vi "Dashboard Main.vi"() -> ()   [LabVIEW 2020]
uses:
  <vilib>/event_ctls.llb/eventvkey.ctl
  <vilib>/Rock Robotics/Network Tables/NT Read Boolean.vi
  <vilib>/Rock Robotics/WPI/Dashboard/WPI_DashboardLogging Global.vi
panel:
  out "Background":bool
  in  "Camera Settings Right":T1={"Frame Rate"=30, "Compression"=30, "Size"=1, "DB Camera Config"=FALSE} {"Frame Rate" scale=1.0..30.0; "Compression" scale=100.0..-1.0; "Size" items=["640x480", "320x240", "160x120"]}
  in  "Camera Name Right":string(combo)="No Camera Selection"
  out "Camera Perf":string
  in  "Camera Settings":T1={"Frame Rate"=30, "Compression"=30, "Size"=1, "DB Camera Config"=FALSE} {"Frame Rate" scale=1.0..30.0; "Compression" scale=100.0..-1.0; "Size" items=["640x480", "320x240", "160x120"]}
  in  "TCP":refnum<k5>
  in  "Rec Mode":enum32{"Stop", "Record", "Playback"}(radio)
  out "Robot IP":string
  out "Image Message":string="Timeout in Camera Communications"
  in  "Dashboard Tab":T2(tab)
  out "Shelf":bool
  in  "Select Auto":string(combo)="Select Autonomous ..."
  out "NT Connection":bool
  out "JS1 Z":dbl(slide) scale=-1.0..1.0 scale format="%#_2e"
  out "JS1 Graph":cluster{"X":dbl, "Y":dbl}[](graph)
  out "JS1 Buttons":T3
  out "JS2 Z":dbl(slide) scale=-1.0..1.0 scale format="%#_2e"
  out "JS2 Graph":cluster{"X":dbl, "Y":dbl}[](graph)
  out "JS2 Buttons":T3
  out "Mode":T4(ring)=enum."Auto Disabled"
  out "Right Camera Perf":cluster{"Bandwidth (Mbps)":dbl, "FPS":dbl}
  out "Moving\nto Target":bool
  out "At Target":bool
  out "Arm \nOverride":bool
  out "Top":bool
  out "Middle":bool
  out "Bottom":bool
  out "Game\nPiece":bool
  out "Speed Modifer":dbl
  out "Reverse":bool
  out "Current Action":string
  out "LiftDmd":dbl
  out "ExtendDmd":dbl
  out "Floor":bool
  out "Camera Image Right":T5(plugin-control)
  in  "DB/String 9":string
  in  "DB/String 8":string
  in  "DB/String 7":string
  in  "DB/String 6":string
  in  "DB/String 5":string
  in  "DB/String 4":string
  in  "DB/String 3":string
  in  "DB/String 2":string
  in  "DB/String 1":string
  in  "DB/String 0":string
  in  "DB/Slider 0":dbl(slide) scale=0.0..5.0
  in  "DB/Slider 1":dbl(slide) scale=0.0..5.0
  in  "DB/Slider 2":dbl(slide) scale=0.0..5.0
  in  "DB/Slider 3":dbl(slide) scale=0.0..5.0
  out "DB/LED 3":bool
  out "DB/LED 2":bool
  out "DB/LED 1":bool
  out "DB/LED 0":bool
  in  "DB/Button 3":bool
  in  "DB/Button 2":bool
  in  "DB/Button 1":bool
  in  "DB/Button 0":bool caption="New Name"
  in  "Test Slider":dbl(slide) scale=0.0..100.0 scale format="%#_3g"
  in  "On/Off":bool caption="Solenoid"
  in  "Test Name":u16(ring) items=["Select the test to run..."]
  in  "Test Tree":string(tree)
  in  "Motor":cluster{"Value":dbl, "Enable":bool} {"Value" scale=-1.0..1.0 scale format="%#_3g"}
  out "Progress":T6 {"Test Progress" scale=0.0..100.0}
  in  "Rev/Fwd":cluster{"Forward":bool, "Reverse":bool}
  in  "Test Ring":u16(ring) items=["Monochrome", "Color"]
  in  "CheckList":i32(listbox)
  out "Tree":string(tree)
  out "Camera Image":T5(plugin-control)
  in  "Camera Name":string(combo)="No Camera Selection"
  # "HW"
  # "HW"
  # "Joysticks"
  # "This tab is a great place for autonomous settings and robot-specific values.\nPlace controls and indicators inside this tab and match name to\nDashboard Variables on robot. You can also delete this comment."
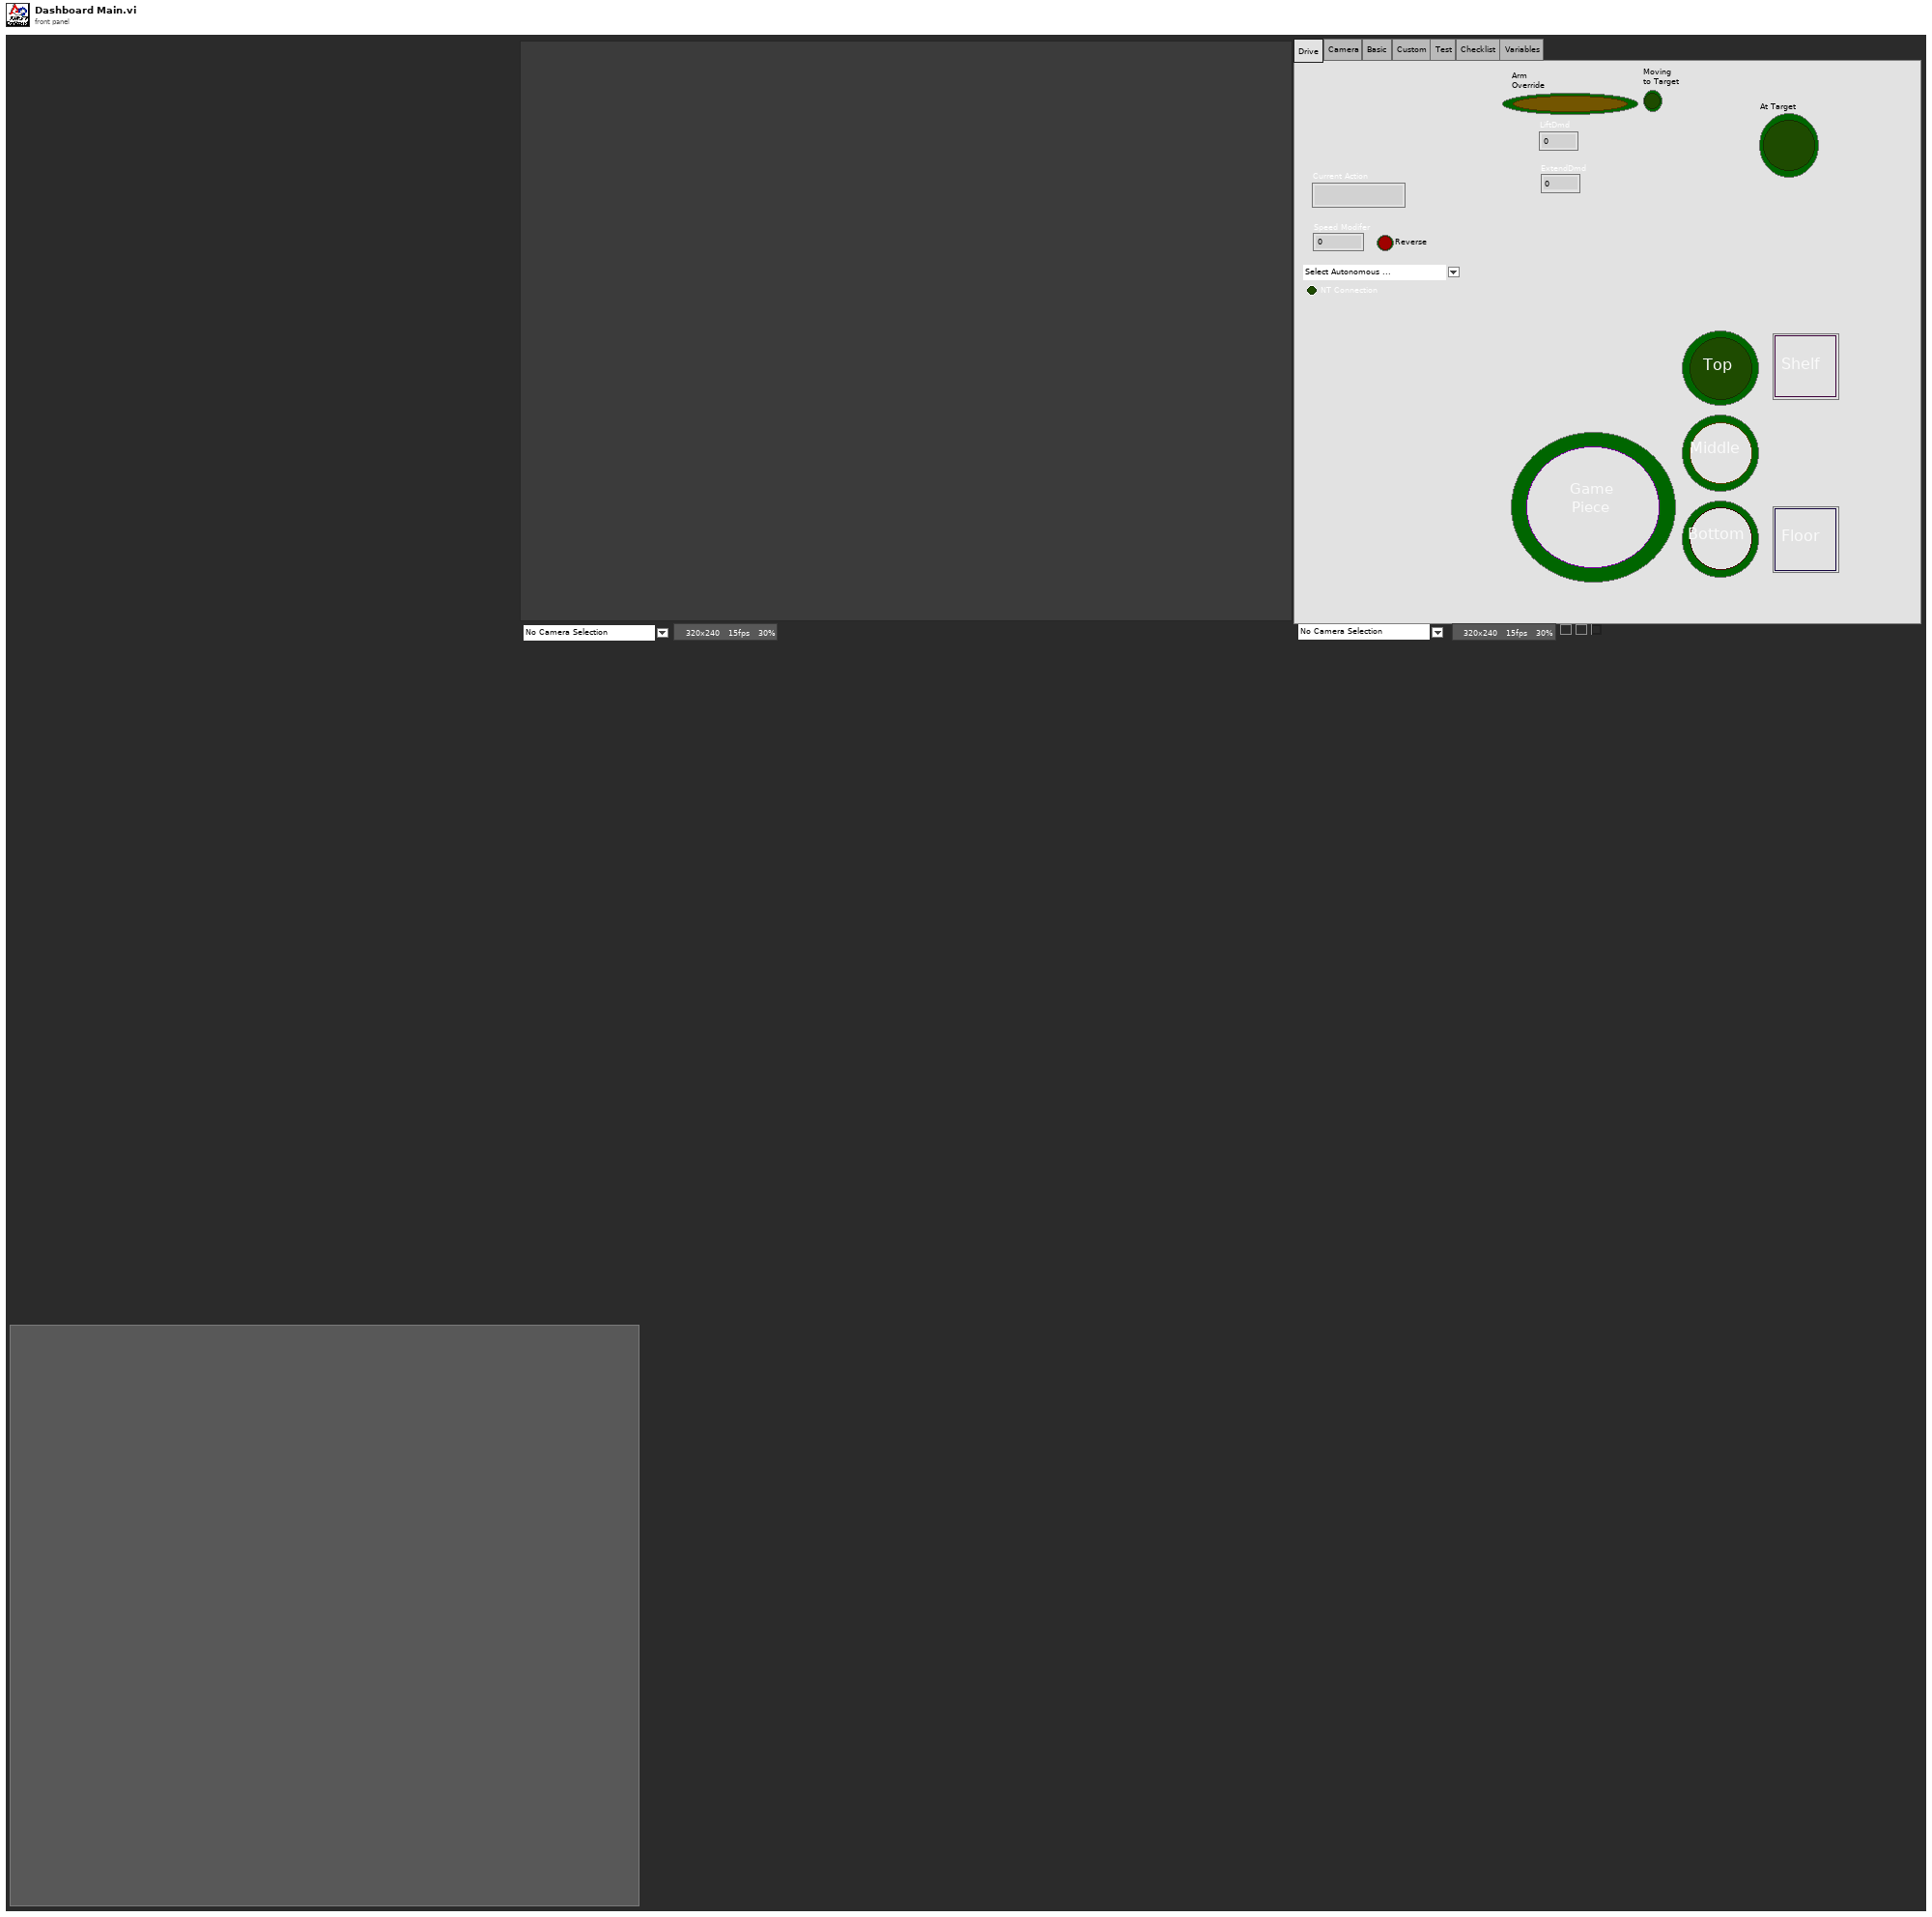
[diagram p1: front panel]
types:
  T1 = cluster{"Frame Rate":i32, "Compression":i32, "Size":u16, "DB Camera Config":bool}
  T2 = enum32{"Drive", "Camera", "Basic", "Custom", "Test", "Checklist", "Variables"}
  T3 = cluster{bool, bool, bool, bool, bool, bool, bool, bool, bool, bool, bool, bool}
  T4 = enum8{"Tele-Op Disabled", "Tele-Op Enabled", "Auto Disabled", "Auto Enabled", "Test Disabled", "Test Enabled", "Disconnected", "No Code", "E-Stop"}
  T5 = typedef "IMAQ Image.ctl" = refnum<image>
  T6 = cluster{"Test Progress":u8, "Test Progress Text":string}
  T7 = cluster{"Save Path":path, "Interval (s)":dbl, "Keep":i32}
  T8 = enum32{"Drive", "Camera", "Basic", "Custom", "Test", "Commands", "Checklist", "Variables"}
  T9 = typedef "Image Type" = u32
  T10 = cluster{"Error Strings":string, "Disable Counts":cluster{u16, u16}, "Rail Faults":cluster{u16, u16, u16}, "Robot IP":string, "DB Mode":u8, "Event Info":cluster{"Name":string, "Type":u8, "Number":u16, "Replay":u8}}
  T11 = cluster{"Storage":cluster{"Disk Free":u64, "RAM Block":u32, "RAM free":u32}, "CPU Utilization":cluster{"CPU % ISR":sgl, "CPU % Time Crit":sgl, "CPU % Timed Str":sgl, "CPU % High":sgl, "CPU % Above":sgl, "CPU % Normal":sgl, "CPU % Low":sgl}, "CAN":cluster{"% Bus Utilization":sgl, "Bus Off Cnt":u32, "TX_FIFO Full Cnt":u32, "Receive Error Cnt":u8, "Transmit Error Cnt":u8}, "HID":cluster{"HID Outputs":u32, "Rumble Low":u16, "Rumble High":u16}[]}
  T12 = cluster{"Status bits":cluster{"Test Mode":bool, "Autonomous":bool, "Enabled":bool, "Code Start":bool, "Brownout":bool, "Reserved 2":bool, "Reserved 3":bool, "E-Stop":bool}, "Code Trace":cluster{"Disabled":bool, "TeleOp":bool, "Auto":bool, "Test":bool}, "Controller Type":enum16{"unknown", "cRIO", "roboRio"}, "Code?":enum16{"unknown", "noCode", "code"}, "Battery V":dbl}
  T13 = cluster{"Control Bits":cluster{"TestMode":bool, "Autonomous":bool, "Enabled":bool, "FMS Present":bool, bool, bool, bool, "E-Stop":bool}, "Team Station ":u8, "Countdown":sgl, "Joystick Values":cluster{"Axes":dbl[], "Buttons":bool[], "POVs":i16[]}[]}
  T14 = cluster{"Axes":dbl[], "Buttons":bool[], "POVs":i16[]}[]
  T15 = cluster{"Axes":dbl[], "Buttons":bool[], "POVs":i16[]}
  T16 = cluster{"Buttons[0]":bool, "Buttons[1]":bool, "Buttons[2]":bool, "Buttons[3]":bool, "Buttons[4]":bool, "Buttons[5]":bool, "Buttons[6]":bool, "Buttons[7]":bool, "Buttons[8]":bool, "Buttons[9]":bool, "Buttons[10]":bool, "Buttons[11]":bool}
  T17 = cluster{"Camera Image":refnum<vi>, "Dashboard Tab":refnum<vi>, "Background":refnum<vi>, "Rec Mode":refnum<vi>, "Test Slider":refnum<vi>, "On/Off ":refnum<vi>, "Test Ring":refnum<vi>, "Rev/Fwd":refnum<vi>, "Test Name":refnum<vi>, "Motor":refnum<vi>, "Progress":refnum<vi>, "CheckList":refnum<vi>, "Tree":refnum<vi>, "Test Tree":refnum<vi>, "Camera Settings":refnum<vi>, "Camera Name":refnum<vi>, "Camera Perf":refnum<vi>, "Camera Settings Right":refnum<vi>, "Camera Name Right":refnum<vi>, "Camera Image Right":refnum<vi>}
  T18 = cluster{"Global Rectangle":i32[], "Contours":cluster{"Contour Type":u32, "ROI Type":u32, "Points":i32[]}[]}
  T19 = cluster{"Camera Name":string, string, "Saved DB Images Info":cluster{"Save Path":path, "Interval (s)":dbl, "Keep":i32}}
  T20 = cluster{"Camera Name Right":string, string, "Saved DB Images Info":cluster{"Save Path":path, "Interval (s)":dbl, "Keep":i32}}
  T21 = cluster{"Operation":enum16{"Update", "Clear"}, "Color Box":u32}[]
  T22 = typedef "eventvkey.ctl" = enum16{"ASCII", "Enter", "Return", "Shift", "Ctrl", "Alt", "Cmd", "Opt", "Caps", "NumLock", "Clear", "Break", "Up", "Down", "Left", "Right", "Insert", "Delete", "Home", "End", "PageUp", "PageDown", "Escape", "Help", "Pause", "ScrollLock", "F1", "F2", "F3", "F4", "F5", "F6", "F7", "F8", "F9", "F10", "F11", "F12", "F13", "F14", "F15", "F16", "F17", "F18", "F19", "F20", "F21", "F22", "F23", "F24", "Play", "VolumeUp", "VolumeDown", "Mute", "Two Byte Char"}
  T23 = cluster{"Image Size":bool, "Image Type":bool, "Pixel Value":bool, "ROI Information":bool, "Zoom Factor":bool}
  T24 = cluster{"Operation":enum16{"Update", "Clear"}, "Color Box":u32}
  T25 = cluster{"Shift":bool, "Ctrl":bool, "Alt":bool, "Cmd":bool, "Opt":bool}
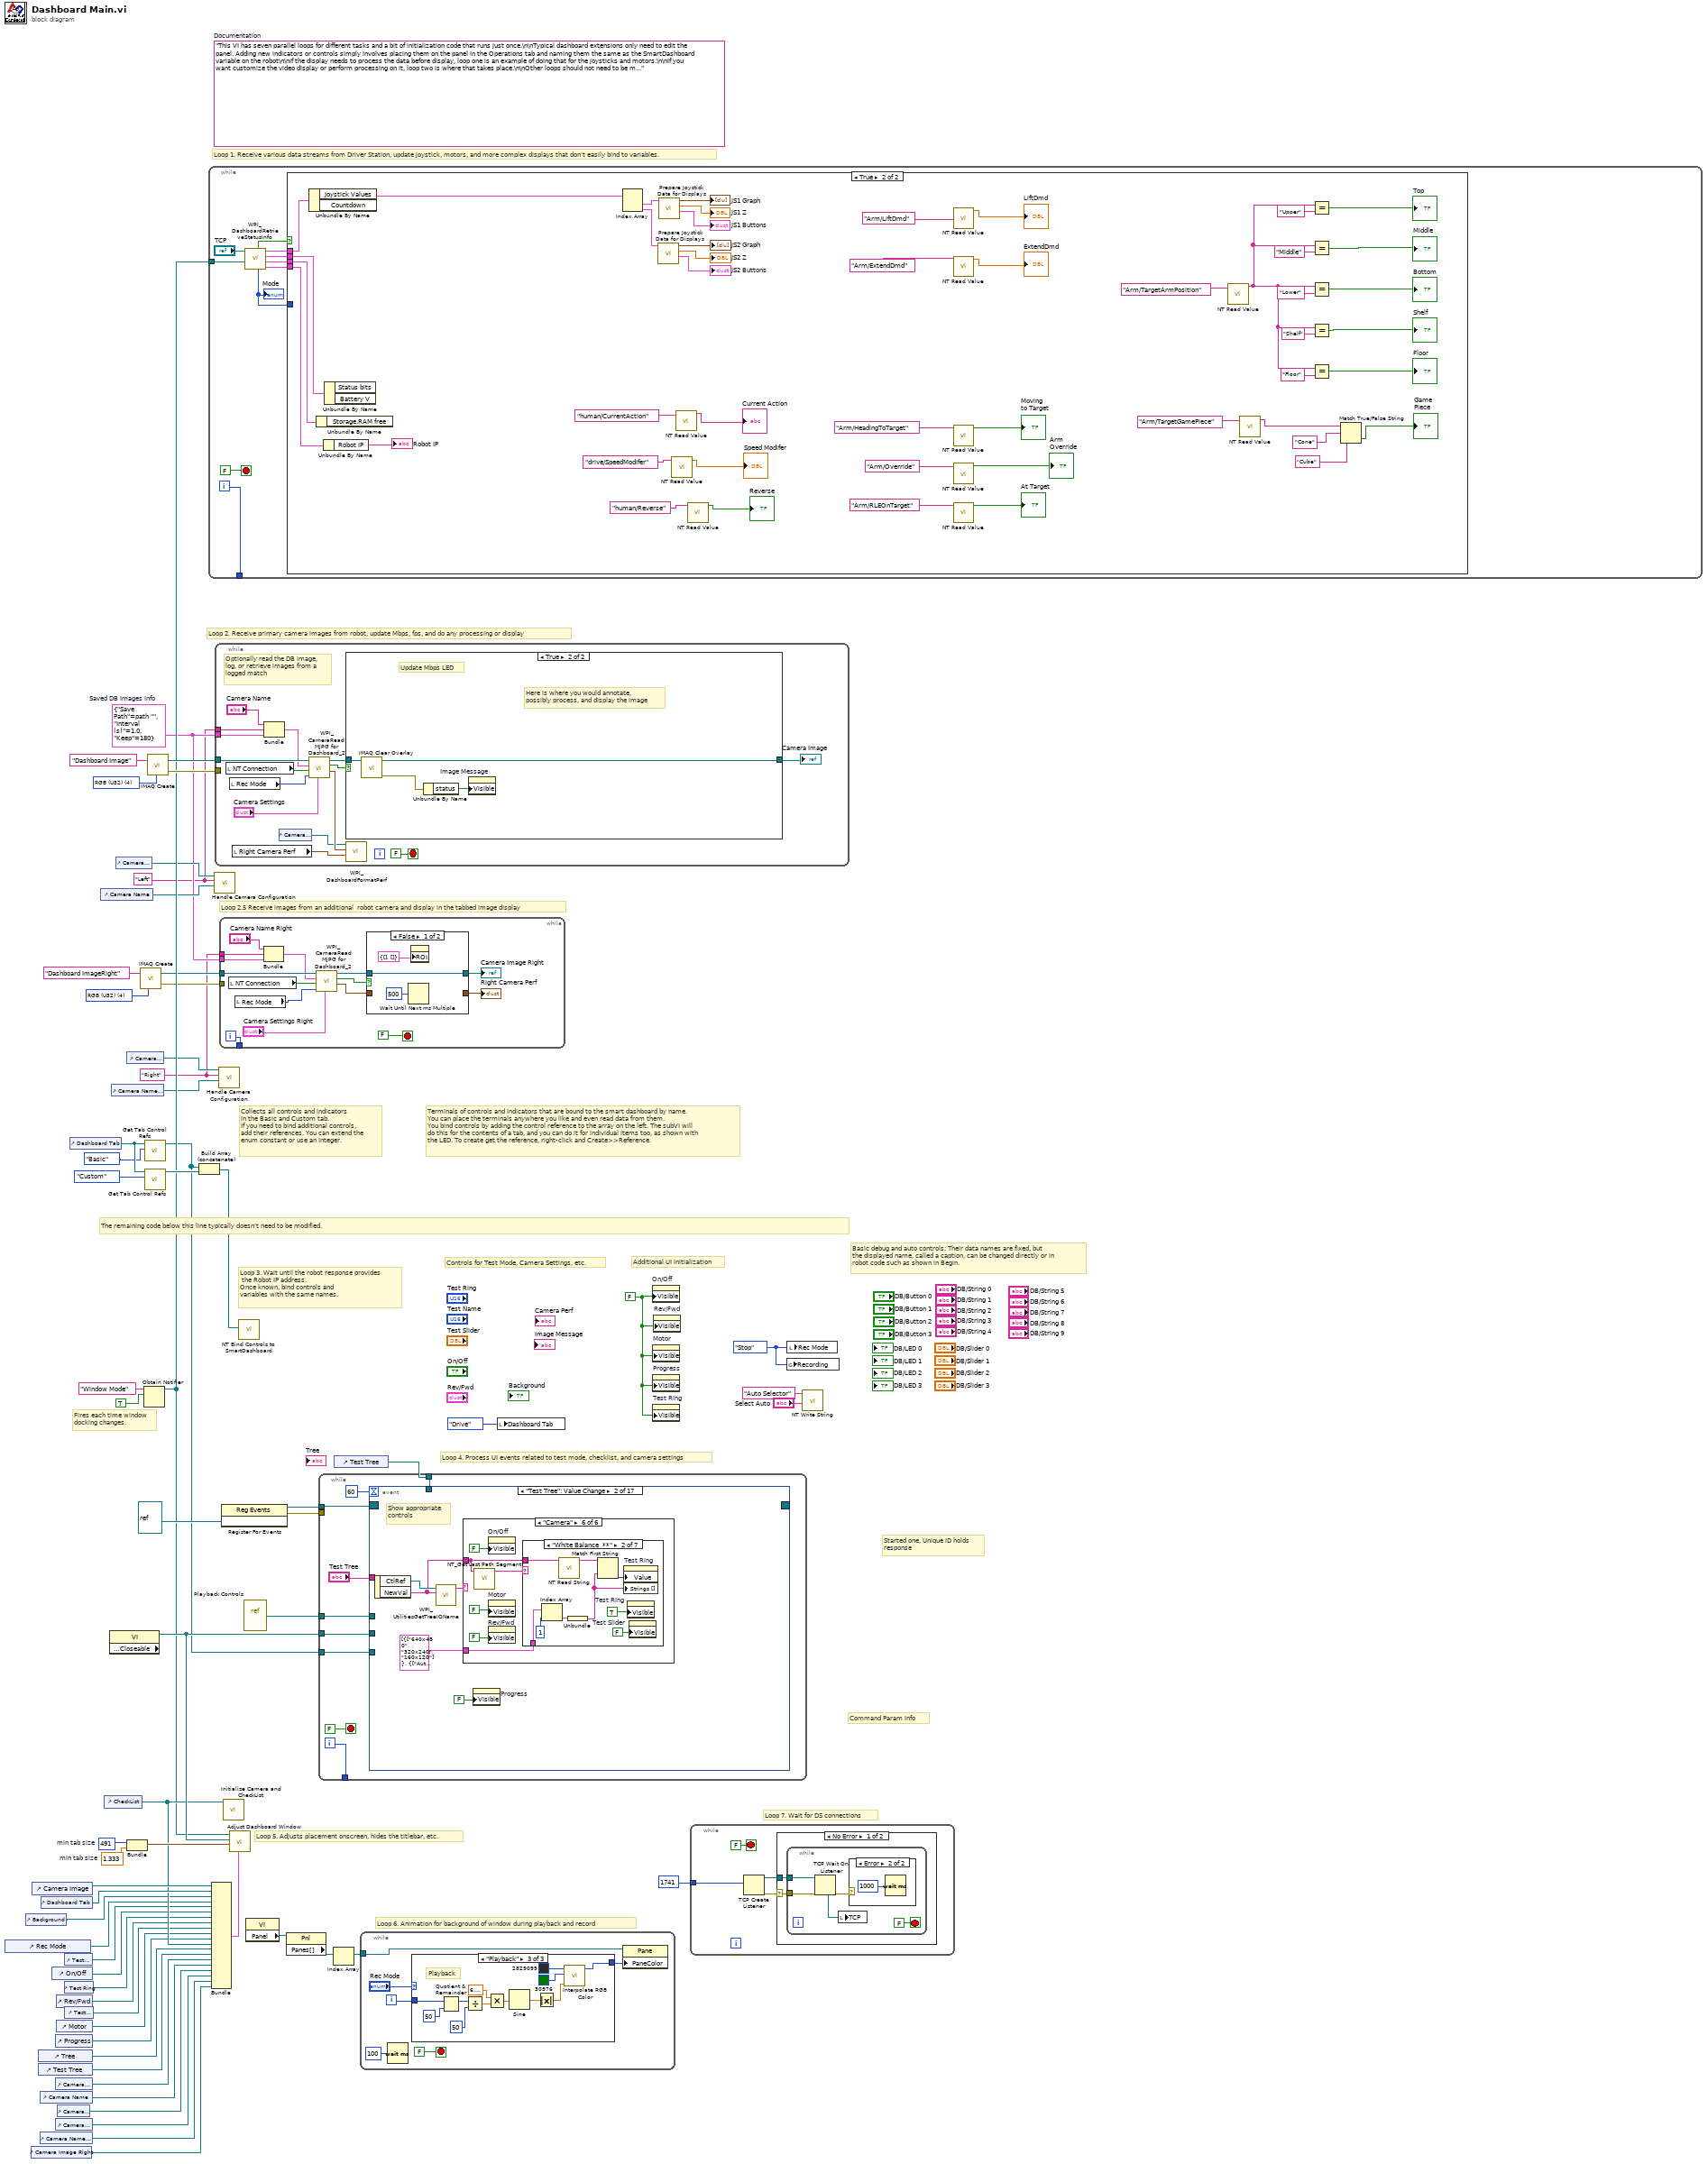
[diagram p0: block diagram]
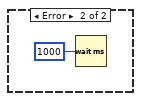
[diagram p4: hidden frame]
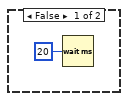
[diagram p5: hidden frame]
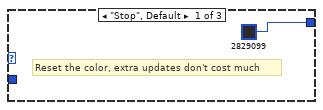
[diagram p6: hidden frame]
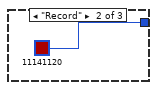
[diagram p7: hidden frame]
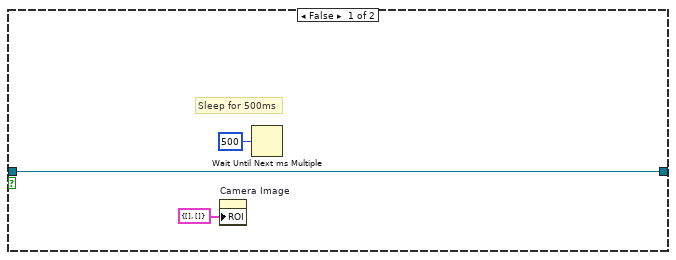
[diagram p8: hidden frame]
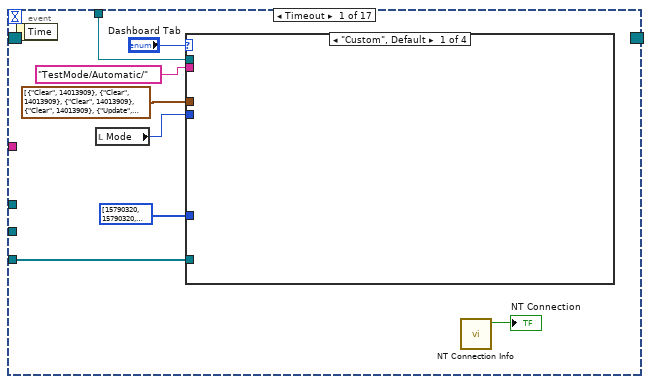
[diagram p9: hidden frame]
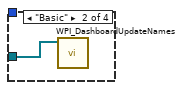
[diagram p10: hidden frame]
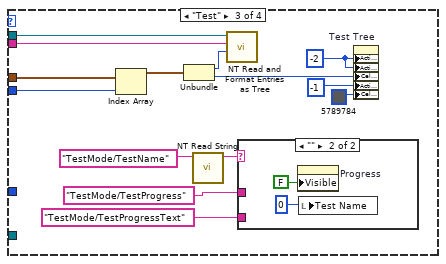
[diagram p11: hidden frame]
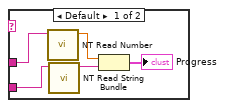
[diagram p12: hidden frame]
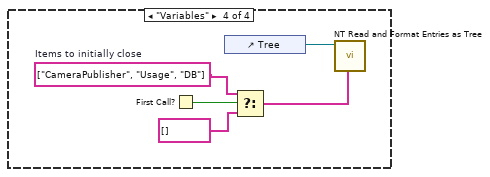
[diagram p13: hidden frame]
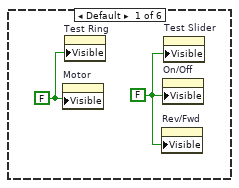
[diagram p14: hidden frame]
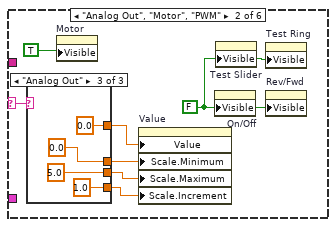
[diagram p15: hidden frame]
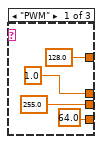
[diagram p16: hidden frame]
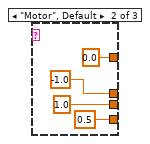
[diagram p17: hidden frame]
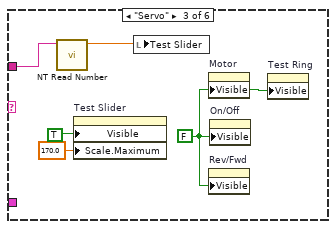
[diagram p18: hidden frame]
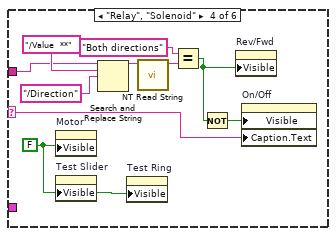
[diagram p19: hidden frame]
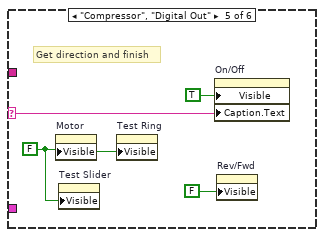
[diagram p20: hidden frame]
diagram:
  w4 = T7 {"Save Path"=path "", "Interval (s)"=1.0, "Keep"=180}  # Saved DB Images Info
  w3 = "Right"
  w2 = "Left"
  w14 = T9 4 items=["Grayscale (U8)", "Grayscale (I16)", "Grayscale (SGL)", "Complex (CSG)", "RGB (U32)", "HSL (U32)", "RGB (U64)"] ("Image Type")
  w42 = 491  # min tab size
  w41 = 1.333  # min tab size
  w49 = enum32{"Stop", "Record", "Playback"}."Stop" ("Rec Mode")
  w27 = FALSE ("Visible")
  (unwired) "This VI has seven parallel loops for different tasks and a bit of initialization code that runs just once.\n\nTypical dashboard extensions only need to edit the panel. Adding new indicators or controls simply involves placing them on the panel in the Operations tab and naming them the same as the SmartDashboard variable on the robot\n\nIf the display needs to process the data before display, loop one is an example of doing that for the joysticks and motors.\n\nIf you want customize the video display or perform processing on it, loop two is where that takes place.\n\nOther loops should not need to be modified. They are pretty standard, and document the task they perform."  # Documentation
  w63 = T9 4 items=["Grayscale (U8)", "Grayscale (I16)", "Grayscale (SGL)", "Complex (CSG)", "RGB (U32)", "HSL (U32)", "RGB (U64)"] ("Image Type")
  # "Loop 2.5 Receive images from an additional  robot camera and display in the tabbed image display"
  # "Command Param Info"
  # "Started one, Unique ID holds\nresponse"
  # "Loop 7. Wait for DS connections"
  # "Basic debug and auto controls: Their data names are fixed, but\nthe displayed name, called a caption, can be changed directly or in\nrobot code such as shown in Begin."
  # "Controls for Test Mode, Camera Settings, etc."
  # "Additional UI Initialization"
  # "Loop 6. Animation for background of window during playback and record"
  # "Fires each time window\ndocking changes."
  # "Collects all controls and indicators\nin the Basic and Custom tab.\nIf you need to bind additional controls,\nadd their references. You can extend the\nenum constant or use an integer."
  # "The remaining code below this line typically doesn't need to be modified."
  # "Loop 4. Process UI events related to test mode, checklist, and camera settings"
  # "Terminals of controls and indicators that are bound to the smart dashboard by name.\nYou can place the terminals anywhere you like and even read data from them.\nYou bind controls by adding the control reference to the array on the left. The subVI will\ndo this for the contents of a tab, and you can do it for individual items too, as shown with\nthe LED. To create get the reference, right-click and Create>>Reference."
  # "Loop 3. Wait until the robot response provides\n the Robot IP address.\nOnce known, bind controls and\nvariables with the same names."
  # "Loop 5. Adjusts placement onscreen, hides the titlebar, etc."
  # "Loop 1. Receive various data streams from Driver Station, update joystick, motors, and more complex displays that don't easily bind to variables."
  # "Loop 2. Receive primary camera images from robot, update Mbps, fps, and do any processing or display"
  n1 = control-ref of="Rec Mode"() -> (w33:refnum<vi>)
  n2 = control-ref of="Background"() -> (w1:refnum<vi>)
  n3 = control-ref of="Camera Image Right"() -> (w7:refnum<vi>)
  n4 = control-ref of="Camera Image"() -> (w44:refnum<vi>)
  n5 = control-ref of="Tree"() -> (w37:refnum<vi>)
  n6 = control-ref of="Test Tree"() -> (w36:refnum<vi>)
  n7 = control-ref of="Camera Name"() -> (w20:refnum<vi>)
  n8 = control-ref of="Camera Name Right"() -> (w8:refnum<vi>)
  n9 = control-ref of="Dashboard Tab"() -> (w43:refnum<vi>)
  n10 = control-ref of="On/Off"() -> (w31:refnum<vi>)
  n11 = control-ref of="Progress"() -> (w28:refnum<vi>)
  n12 = control-ref of="Camera Settings"() -> (w21:refnum<vi>)
  n13 = control-ref of="Camera Settings Right"() -> (w9:refnum<vi>)
  n14 = control-ref of="Rev/Fwd"() -> (w29:refnum<vi>)
  n15 = control-ref of="Motor"() -> (w34:refnum<vi>)
  n16 = control-ref of="Camera Perf"() -> (w19:refnum<vi>)
  n17 = control-ref of="Test Slider"() -> (w32:refnum<vi>)
  n18 = control-ref of="Test Ring"() -> (w30:refnum<vi>)
  n19 = control-ref of="Test Name"() -> (w35:refnum<vi>)
  n20 = control-ref of="Dashboard Tab"() -> (w47:refnum<vi>)
  n21 = control-ref of="Camera Name"() -> (w22:refnum<vi>)
  n22 = control-ref of="CheckList"() -> (w38:refnum<vi>)
  n23 = property class="VI" props=["Front Panel.Closeable"]() -> (reference out=w48:refnum<vi>)  [unwired: 2 in, 2 out]
  n24 = control-ref of="Camera Name Right"() -> (w10:refnum<vi>)
  n25 = control-ref of="Camera Settings"() -> (w23:refnum<vi>)
  n26 = control-ref of="Camera Settings Right"() -> (w11:refnum<vi>)
  n27 = Bundle("min tab size"=w42, "min tab size"=w41) -> (w40:cluster{"min tab size":i32, "min tab size":dbl})  [unwired: 1 in]
  n28 = call "IMAQ Create"("Image Name"="Dashboard ImageRight", "Image Type"=w14) -> ("New Image"=w13:T5, "error out"=w12:errorcluster)  [unwired: 2 in, 1 out]
  n29 = Obtain Notifier(name (unnamed)="Window Mode", notification data type=TRUE) -> (notifier out=w26:refnum<notifier>)  [unwired: 2 in, 2 out]
  n30 = call <vilib>:"Get Tab Control Refs.vi"("Page Index"=T8."Basic" ("Dashboard Tab"), "TabControl in"=w47) -> ("ControlsOnPage"=w18:refnum<vi>[])  [unwired: 9 in]
  n31 = call <vilib>:"Get Tab Control Refs.vi"("Page Index"=T8."Custom" ("Dashboard Tab"), "TabControl in"=w47) -> ("ControlsOnPage"=w46:refnum<vi>[])  [unwired: 9 in]
  n32 = call "IMAQ Create"("Image Name"="Dashboard Image", "Image Type"=w63) -> ("New Image"=w61:T5, "error out"=w60:errorcluster)  [unwired: 2 in, 1 out]
  n33 = Build Array (concatenate)(w18, w46) -> (w45:refnum<vi>[])
  n34 = while {
    tunnel: [w72] -> _
    tunnel: w26 -> [w64]
    i -> [w72]
    stop <- FALSE stop-if-true
    n35 = call <vilib>:"WPI_DashboardRetrieveStatusInfo.vi"("Window Mode Notifier"=w64, "TCP Cnx"="TCP") -> ("Power and Errors"=w67:T10, "Robot Metrics"=w70:T11, "Status Info"=w71:T12, "Control Info"=w68:T13, "Robot Mode"=w66:T4, "Process?"=w69:bool)  [unwired: 4 in]
    "Mode" <- w66
    n36 = case shown="True" w69 {
      tunnel: w71 -> [_ w121]
      tunnel: w70 -> [_ w120]
      tunnel: w68 -> [_ w119]
      tunnel: w67 -> [_ w118]
      tunnel: w66 -> [_ _]
      frame False {
        n37 = Wait (ms)(milliseconds to wait=u32 20) -> ()  [unwired: 1 out]
      }
      frame True {
        n38 = Unbundle By Name(w119) -> ("Joystick Values"=w117:T14)  [unwired: 1 out]
        n39 = Unbundle By Name(w120) -> ()  [unwired: 1 out]
        n40 = Unbundle By Name(w118) -> ("Robot IP"=→"Robot IP":string)
        n41 = Unbundle By Name(w121) -> ()  [unwired: 2 out]
        n42 = Index Array(array=w117) -> (element #1=w116:T15, element #2=w112:T15)  [unwired: 2 in]
        n43 = call "Prepare Joystick Data for Displays.vi"("Joystick Values"=w112) -> ("Buttons"=→"JS2 Buttons":T16, "Z Axis"=→"JS2 Z":dbl, "Cartesian Data"=→"JS2 Graph":cluster{"X axis":dbl, "X axis":dbl}[])  [unwired: 8 in]
        n44 = call "Prepare Joystick Data for Displays.vi"("Joystick Values"=w116) -> ("Buttons"=→"JS1 Buttons":T16, "Z Axis"=→"JS1 Z":dbl, "Cartesian Data"=→"JS1 Graph":cluster{"X axis":dbl, "X axis":dbl}[])  [unwired: 8 in]
        n45 = call-poly <vilib>:"NT Read Value.vi"("name"="drive/SpeedModifer") -> ("value"=→"Speed Modifer":dbl)  [unwired: 8 in, 2 out]
        n46 = call-poly <vilib>:"NT Read Value.vi"("name"="human/CurrentAction") -> ("value"=→"Current Action":string)  [unwired: 8 in, 2 out]
        n47 = call-poly <vilib>:"NT Read Value.vi"("name"="human/Reverse") -> ("value"=→"Reverse":bool)  [unwired: 8 in, 2 out]
        n48 = call-poly <vilib>:"NT Read Value.vi"("name"="Arm/LiftDmd") -> ("value"=→"LiftDmd":dbl)  [unwired: 8 in, 2 out]
        n49 = call-poly <vilib>:"NT Read Value.vi"("name"="Arm/ExtendDmd") -> ("value"=→"ExtendDmd":dbl)  [unwired: 8 in, 2 out]
        n50 = call-poly <vilib>:"NT Read Value.vi"("name"="Arm/HeadingToTarget") -> ("value"=→"Moving\nto Target":bool)  [unwired: 8 in, 2 out]
        n51 = call-poly <vilib>:"NT Read Value.vi"("name"="Arm/Override") -> ("value"=→"Arm \nOverride":bool)  [unwired: 8 in, 2 out]
        n52 = call-poly <vilib>:"NT Read Value.vi"("name"="Arm/RLEOnTarget") -> ("value"=→"At Target":bool)  [unwired: 8 in, 2 out]
        n53 = call-poly <vilib>:"NT Read Value.vi"("name"="Arm/TargetArmPosition") -> ("value"=w90:string)  [unwired: 8 in, 2 out]
        n54 = call-poly <vilib>:"NT Read Value.vi"("name"="Arm/TargetGamePiece") -> ("value"=w83:string)  [unwired: 8 in, 2 out]
        n55 = Equal?(x=w90, y="Upper") -> (x = y?=→"Top":bool)
        n56 = Equal?(x=w90, y="Middle") -> (x = y?=→"Middle":bool)
        n57 = Equal?(x=w90, y="Lower") -> (x = y?=→"Bottom":bool)
        n58 = Equal?(x=w90, y="Shelf") -> (x = y?=→"Shelf":bool)
        n59 = Equal?(x=w90, y="Floor") -> (x = y?=→"Floor":bool)
        n60 = Match True/False String(2:"Cube" ("false string"), 3:"Cone" ("true string"), 4:w83) -> (0:→"Game\nPiece":bool)  [unwired: 1 out]
      }
    }
  }
  n61 = Bundle("Camera Image"=w44, "Dashboard Tab"=w43, "Background"=w1, "Rec Mode"=w33, "Test Slider"=w32, "On/Off"=w31, "Test Ring"=w30, "Rev/Fwd"=w29, "Test Name"=w35, "Motor"=w34, "Progress"=w28, "CheckList"=w38, "Tree"=w37, "Test Tree"=w36, "Camera Settings"=w21, "Camera Name"=w20, "Camera Perf"=w19, "Camera Settings Right"=w9, "Camera Name Right"=w8, "Camera Image Right"=w7) -> (w39:T17)  [unwired: 1 in]
  n62 = call "Handle Camera Configuration.vi"("CameraNameRef"=w22, "Display Name"=w2, "ClusterRef"=w23) -> ()  [unwired: 9 in]
  n63 = while {
    tunnel: w61 -> [w135]
    tunnel: w60 -> [_]
    tunnel: w4 -> [w128]
    tunnel: w2 -> [w125]
    stop <- FALSE stop-if-true
    # "Optionally read the DB image,\nlog, or retrieve images from a\nlogged match"
    n64 = local read "NT Connection"() -> (w129:bool)
    n65 = local read "Rec Mode"() -> (w132:enum32{"Stop", "Record", "Playback"})
    n66 = local read "Right Camera Perf"() -> (w123:cluster{"Bandwidth (Mbps)":dbl, "FPS":dbl})
    n67 = Bundle("Camera Name"="Camera Name", w125, "Saved DB Images Info"=w128) -> (w127:T19)  [unwired: 1 in]
    n68 = control-ref of="Camera Perf"() -> (w122:refnum<vi>)
    n69 = call <vilib>:"WPI_CameraRead MJPG for Dashboard_2.vi"("Camera Settings"="Camera Settings", "Rec Mode"=w132, "NT Connection"=w129, "Capture Info"=w127, "Image in"=w135) -> ("perf info"=w124:cluster{"Bandwidth (Mbps)":dbl, "fps":dbl}, "Active"=w133:bool, "Image\\ out"=w134:T5)  [unwired: 4 in]
    n70 = case shown="True" w133 {
      tunnel: w134 -> [w138 w141]
      tunnel: [w138 w140] -> w130
      frame False {
        # "Sleep for 500ms"
        n71 = property on="Camera Image" class="ImageControl"("ROI"=T18 {"Global Rectangle"=[], "Contours"=[]}) -> ()  [unwired: 2 in, 2 out]
        n72 = Wait Until Next ms Multiple(millisecond multiple=u32 500) -> ()  [unwired: 1 out]
      }
      frame True {
        # "Here is where you would annotate,\npossibly process, and display the image"
        # "Update Mbps LED"
        n73 = call "IMAQ Clear Overlay"("Image"=w141) -> ("error out"=w142:errorcluster, "Image Out"=w140:T5)  [unwired: 2 in, 7 out]
        n74 = Unbundle By Name(w142) -> ("status"=w143:bool)
        n75 = property on="Image Message" class="Str"("Visible"=w143) -> ()  [unwired: 2 in, 2 out]
      }
    }
    "Camera Image" <- w130
    n76 = call <vilib>:"WPI_DashboardFormatPerf.vi"("Right Camera Perf"=w123, "Performance"=w124, "String in"=w122) -> ()  [unwired: 9 in]
  }
  n77 = call "Handle Camera Configuration.vi"("CameraNameRef"=w10, "Display Name"=w3, "ClusterRef"=w11) -> ()  [unwired: 9 in]
  n78 = while {
    tunnel: w13 -> [w158]
    tunnel: w12 -> [_]
    tunnel: [w153] -> _
    tunnel: w4 -> [w149]
    tunnel: w3 -> [w146]
    i -> [w153]
    stop <- FALSE stop-if-true
    n79 = local read "NT Connection"() -> (w150:bool)
    n80 = local read "Rec Mode"() -> (w157:enum32{"Stop", "Record", "Playback"})
    n81 = Bundle("Camera Name Right"="Camera Name Right", w146, "Saved DB Images Info"=w149) -> (w148:T20)  [unwired: 1 in]
    n82 = call <vilib>:"WPI_CameraRead MJPG for Dashboard_2.vi"("Camera Settings"="Camera Settings Right", "Rec Mode"=w157, "NT Connection"=w150, "Capture Info"=w148, "Image in"=w158) -> ("perf info"=w144:cluster{"Bandwidth (Mbps)":dbl, "fps":dbl}, "Active"=w152:bool, "Image\\ out"=w155:T5)  [unwired: 4 in]
    n83 = case shown="False" w152 {
      tunnel: w155 -> [w160 w163]
      tunnel: [w160 w163] -> w151
      tunnel: [_ w162] -> w145
      tunnel: w144 -> [_ w162]
      frame False {
        n84 = Wait Until Next ms Multiple(millisecond multiple=u32 500) -> ()  [unwired: 1 out]
        n85 = property on="Camera Image Right" class="ImageControl"("ROI"=T18 {"Global Rectangle"=[], "Contours"=[]}) -> ()  [unwired: 2 in, 2 out]
      }
      frame True {
      }
    }
    "Camera Image Right" <- w151
    "Right Camera Perf" <- w145
  }
  n86 = register-events(refnum<vi> refnum) -> (reference out=w52:refnum<event-registration>, error out=w51:errorcluster)  [unwired: 2 in]
  n87 = call "Initialize Camera and CheckList.vi"("ListBox in"=w38) -> ()  [unwired: 11 in]
  n88 = call "Adjust Dashboard Window.vi"("Sizing Refnums"=w39, "Size Constraints"=w40, "VI"=w48, "WIn Mode"=w26) -> ()  [unwired: 8 in]
  n89 = call <vilib>:"NT Bind Controls to SmartDashboard.vi"("Bound Control Refs"=w45) -> ()  [unwired: 11 in]
  n90 = vi-ref "Playback Controls.vi"() -> (w53:refnum<vi>)
  n91 = property class="VI"() -> ("Panel"=w55:refnum<vi>)  [unwired: 2 in, 2 out]
  n92 = property class="Pnl"(reference=w55) -> ("Panes[]"=w56:refnum<vi>[])  [unwired: 1 in, 2 out]
  n93 = Index Array(array=w56) -> (element=w54:refnum<vi>)  [unwired: 1 in]
  n94 = control-ref of="Test Tree"() -> (w57:refnum<vi>)
  n95 = while {
    tunnel: [w169] -> _
    tunnel: w57 -> [w168]
    tunnel: w53 -> [w167]
    tunnel: w52 -> [w166]
    tunnel: w51 -> [_]
    tunnel: w48 -> [w165]
    tunnel: w18 -> [w164]
    i -> [w169]
    stop <- FALSE stop-if-true
    n96 = event shown="[1] \"Test Tree\": Value Change" {
      selector: w166 -> [_ _ _ _ _ _ _ _ _ _ _ _ _ _ _ _ _]
      dyn-events: [_ _ _ _ _ _ _ _ _ _ _ _ _ w374 _ _ _] -> _
      timeout: u32 60 ("milliseconds to wait") -> [_ _ _ _ _ _ _ _ _ _ _ _ _ _ _ _ _]
      tunnel: w168 -> [w179 _ _ _ _ _ _ _ _ _ _ _ _ _ _ _ _]
      tunnel: "Test Tree" -> [_ _ _ _ _ _ _ _ w347 w354 w355 w358 w365 _ _ _ _]
      tunnel: w167 -> [_ _ _ _ _ _ _ _ _ _ _ _ _ w376 _ w391 _]
      tunnel: w165 -> [_ _ _ _ _ _ _ _ _ _ _ _ _ w372 _ _ _]
      tunnel: w164 -> [w174 _ _ _ _ _ _ _ _ _ _ _ _ _ _ _ _]
      event Timeout {
        n97 = event-data() -> ()  [unwired: 1 in, 1 out]
        n98 = local read "Mode"() -> (w177:T4)
        n99 = case shown="\"Custom\", Default" "Dashboard Tab" {
          tunnel: w179 -> [_ _ w195 _]
          tunnel: "TestMode/Automatic/" ("Name Pattern") -> [_ _ w194 _]
          tunnel: T21 [{"Operation"=enum."Clear", "Color Box"=14013909}, {"Operation"=enum."Clear", "Color Box"=14013909}, {"Operation"=enum."Clear", "Color Box"=14013909}, {"Operation"=enum."Clear", "Color Box"=14013909}, {"Operation"=enum."Update", "Color Box"=14013909}, {"Operation"=enum."Update", "Color Box"=16777215}, {"Operation"=enum."Clear", "Color Box"=14013909}, {"Operation"=enum."Clear", "Color Box"=14013909}, {"Operation"=enum."Clear", "Color Box"=14013909}] -> [_ _ w187 _]
          tunnel: w177 -> [_ _ w186 _]
          tunnel: u32[] [15790320, 15790320, 15790320, 15790320, 16777215, 16777215, 15790320, 15790320, 15790320] -> [_ _ _ _]
          tunnel: w174 -> [_ w181 _ _]
          frame "Custom", Default {
          }
          frame "Basic" {
            n100 = call <vilib>:"WPI_DashboardUpdateNames.vi"("Controls on Tab"=w181) -> ()  [unwired: 11 in]
          }
          frame "Test" {
            w193 = -2 ("Active Item:Row Number")
            n101 = Index Array(array=w187, index=w186) -> (element=w188:T24)
            n102 = Unbundle(w188) -> ("Operation"=w189:enum16{"Update", "Clear"}, "Color Box"=w190:u32)
            n103 = call <vilib>:"NT Read String.vi"("name"="TestMode/TestName" ("Name")) -> ("value"=w184:string)  [unwired: 8 in, 2 out]
            n104 = call <vilib>:"NT Read and Format Entries as Tree.vi"("Operation"=w189, "Name Pattern"=w194, "Tree Refnum"=w195) -> ()  [unwired: 7 in, 2 out]
            n105 = case shown="\"\"" w184 {
              tunnel: "TestMode/TestProgress" ("Name") -> [w197 _]
              tunnel: "TestMode/TestProgressText" ("Name") -> [w196 _]
              frame Default {
                n106 = call <vilib>:"NT Read Number.vi"("name"=w197) -> ("value"=w198:dbl)  [unwired: 8 in, 2 out]
                n107 = call <vilib>:"NT Read String.vi"("name"=w196) -> ("value"=w199:string)  [unwired: 8 in, 2 out]
                n108 = Bundle("value"=w198, "value"=w199) -> (→"Progress":cluster{"value":dbl, "value":string})  [unwired: 1 in]
              }
              frame "" {
                n109 = property on="Progress" class="Clust (strict)"("Visible"=FALSE) -> ()  [unwired: 2 in, 2 out]
                n110 = local write "Test Name"(u16 0) -> ()
              }
            }
            n111 = property on="Test Tree" class="Tree (strict)"("Active Item Row Number"=w193, "ActiveColNum"=w193, "CellBG"=w190, "Active Item Row Number"=-1 ("Active Item:Row Number"), "CellBG"=u32 5789784 ("Color Box")) -> ()  [unwired: 2 in, 2 out]
          }
          frame "Variables" {
            w205 = string[] ["CameraPublisher", "Usage", "DB"]  # Items to initially close
            n112 = First Call?() -> (First Call?: T/F=w206:bool)
            n113 = control-ref of="Tree"() -> (w207:refnum<vi>)
            n114 = Select(t=w205, s=w206, f=string[] []) -> (s? t:f=w203:string[])
            n115 = call <vilib>:"NT Read and Format Entries as Tree.vi"("Tags to  Close"=w203, "Tree Refnum"=w207) -> ()  [unwired: 8 in, 2 out]
          }
        }
        n116 = call <vilib>:"NT Connection Info.vi"() -> ("Connected"=→"NT Connection":bool)  [unwired: 11 in]
      }
      event "Test Tree": Value Change {
        # "Show appropriate\ncontrols"
        n117 = event-data() -> ("CtlRef"=w211:refnum<vi>, "NewVal"=w209:string)  [unwired: 1 in]
        n118 = call <vilib>:"WPI_UtilitiesGetTreeIOName.vi"("NewVal"=w209, "TreeControl in"=w211) -> ("I/O Name"=w212:string)  [unwired: 9 in]
        n119 = case shown="\"Camera\"" w212 {
          selector: w212 -> [_ w219 _ w241 w250 _]
          tunnel: w209 -> [_ _ w238 w240 _ w257]
          tunnel: cluster{string[]}[] [{["640x480", "320x240", "160x120"]}, {["Auto", "Fixed indoor", "Fixed outdoor 1", "Fixed outdoor 2", "Fixed fluorescent 1", "Fixed fluorescent 2", "Hold current"]}, {["Auto", "Flicker-free 50 Hz", "Flicker-free 60 Hz", "Hold current"]}, {["None", "Prioritize frame rate", "Prioritize image quality"]}, {["Monochrome", "Color"]}] -> [_ _ _ _ _ w256]
          frame Default {
            w214 = FALSE ("Visible")
            w213 = FALSE ("Visible")
            n120 = property on="Motor" class="Clust (strict)"("Visible"=w213) -> ()  [unwired: 2 in, 2 out]
            n121 = property on="Test Ring" class="Ring (strict)"("Visible"=w213) -> ()  [unwired: 2 in, 2 out]
            n122 = property on="Rev/Fwd" class="Clust (strict)"("Visible"=w214) -> ()  [unwired: 2 in, 2 out]
            n123 = property on="On/Off" class="Bool (strict)"("Visible"=w214) -> ()  [unwired: 2 in, 2 out]
            n124 = property on="Test Slider" class="Slide (strict)"("Visible"=w214) -> ()  [unwired: 2 in, 2 out]
          }
          frame "Analog Out", "Motor", "PWM" {
            w220 = FALSE ("Visible")
            n125 = case shown="\"Analog Out\"" w219 {
              tunnel: [1.0 ("Value") -1.0 ("Value") 0.0 ("Value")] -> w218
              tunnel: [255.0 ("Value") 1.0 ("Value") 5.0 ("Value")] -> w217
              tunnel: [128.0 ("Value") 0.0 ("Value") 0.0 ("Value")] -> w216
              tunnel: [64.0 ("Value") 0.5 ("Value") 1.0 ("Value")] -> w215
              frame "PWM" {
              }
              frame "Motor", Default {
              }
              frame "Analog Out" {
              }
            }
            n126 = property on="Motor" class="Clust (strict)"("Visible"=TRUE) -> ()  [unwired: 2 in, 2 out]
            n127 = property on="Value" class="Slide (strict)"("Value"=w216, "Scale.Minimum"=w218, "Scale.Maximum"=w217, "Scale.Increment"=w215) -> ()  [unwired: 2 in, 2 out]
            n128 = property on="On/Off" class="Bool (strict)"("Visible"=w220) -> ()  [unwired: 2 in, 2 out]
            n129 = property on="Test Slider" class="Slide (strict)"("Visible"=w220) -> ()  [unwired: 2 in, 2 out]
            n130 = property on="Test Ring" class="Ring (strict)"("Visible"=w220) -> ()  [unwired: 2 in, 2 out]
            n131 = property on="Rev/Fwd" class="Clust (strict)"("Visible"=w220) -> ()  [unwired: 2 in, 2 out]
          }
          frame "Servo" {
            w236 = FALSE ("Visible")
            n132 = call <vilib>:"NT Read Number.vi"("name"=w238) -> ("value"=w237:dbl)  [unwired: 8 in, 2 out]
            n133 = property on="Test Slider" class="Slide (strict)"("Visible"=TRUE, "Scale.Maximum"=170.0 ("Scale.Range:Maximum")) -> ()  [unwired: 2 in, 2 out]
            n134 = local write "Test Slider"(w237) -> ()
            n135 = property on="Motor" class="Clust (strict)"("Visible"=w236) -> ()  [unwired: 2 in, 2 out]
            n136 = property on="Rev/Fwd" class="Clust (strict)"("Visible"=w236) -> ()  [unwired: 2 in, 2 out]
            n137 = property on="On/Off" class="Bool (strict)"("Visible"=w236) -> ()  [unwired: 2 in, 2 out]
            n138 = property on="Test Ring" class="Ring (strict)"("Visible"=w236) -> ()  [unwired: 2 in, 2 out]
          }
          frame "Relay", "Solenoid" {
            w239 = FALSE ("Visible")
            n139 = property on="Motor" class="Clust (strict)"("Visible"=w239) -> ()  [unwired: 2 in, 2 out]
            n140 = property on="Test Slider" class="Slide (strict)"("Visible"=w239) -> ()  [unwired: 2 in, 2 out]
            n141 = Search and Replace String(input string=w240, search string="/Value  **", replace string="/Direction") -> (result string=w246:string)  [unwired: 5 in, 3 out]
            n142 = property on="Test Ring" class="Ring (strict)"("Visible"=w239) -> ()  [unwired: 2 in, 2 out]
            n143 = call <vilib>:"NT Read String.vi"("name"=w246) -> ("value"=w244:string)  [unwired: 8 in, 2 out]
            n144 = Equal?(x="Both directions", y=w244) -> (x = y?=w242:bool)
            n145 = Not(x=w242) -> (.not. x?=w243:bool)
            n146 = property on="Rev/Fwd" class="Clust (strict)"("Visible"=w242) -> ()  [unwired: 2 in, 2 out]
            n147 = property on="On/Off" class="Bool (strict)"("Visible"=w243, "Caption.Text"=w241) -> ()  [unwired: 2 in, 2 out]
          }
          frame "Compressor", "Digital Out" {
            w249 = FALSE ("Visible")
            # "Get direction and finish"
            n148 = property on="Motor" class="Clust (strict)"("Visible"=w249) -> ()  [unwired: 2 in, 2 out]
            n149 = property on="Test Slider" class="Slide (strict)"("Visible"=w249) -> ()  [unwired: 2 in, 2 out]
            n150 = property on="Test Ring" class="Ring (strict)"("Visible"=w249) -> ()  [unwired: 2 in, 2 out]
            n151 = property on="On/Off" class="Bool (strict)"("Visible"=TRUE, "Caption.Text"=w250) -> ()  [unwired: 2 in, 2 out]
            n152 = property on="Rev/Fwd" class="Clust (strict)"("Visible"=FALSE) -> ()  [unwired: 2 in, 2 out]
          }
          frame "Camera" {
            n153 = call <vilib>:"NT_Get Last Path Segment.vi"("String in"=w257) -> ("String out"=w258:string)  [unwired: 10 in]
            n154 = property on="On/Off" class="Bool (strict)"("Visible"=FALSE) -> ()  [unwired: 2 in, 2 out]
            n155 = property on="Motor" class="Clust (strict)"("Visible"=FALSE) -> ()  [unwired: 2 in, 2 out]
            n156 = property on="Rev/Fwd" class="Clust (strict)"("Visible"=FALSE) -> ()  [unwired: 2 in, 2 out]
            n157 = case shown="\"White Balance  **\"" w258 {
              tunnel: w257 -> [w264 w273 w282 w291 w300 _ w306]
              tunnel: w256 -> [w262 w270 w279 w288 w297 _ _]
              frame "Size  **" {
                n158 = Index Array(array=w262) -> (element=w261:cluster{string[]})  [unwired: 1 in]
                n159 = call <vilib>:"NT Read String.vi"("name"=w264) -> ("value"=w263:string)  [unwired: 8 in, 2 out]
                n160 = Unbundle(w261) -> (w259:string[])
                n161 = Match First String(2:w259, 3:w263) -> (0:w260:i32)  [unwired: 1 out]
                n162 = property on="Test Ring" class="Ring (strict)"("Value"=w260, "Strings []"=w259) -> ()  [unwired: 2 in, 2 out]
                n163 = property on="Test Ring" class="Ring (strict)"("Visible"=TRUE) -> ()  [unwired: 2 in, 2 out]
                n164 = property on="Test Slider" class="Slide (strict)"("Visible"=FALSE) -> ()  [unwired: 2 in, 2 out]
              }
              frame "White Balance  **" {
                n165 = Index Array(array=w270, index=1) -> (element=w271:cluster{string[]})
                n166 = call <vilib>:"NT Read String.vi"("name"=w273) -> ("value"=w272:string)  [unwired: 8 in, 2 out]
                n167 = Unbundle(w271) -> (w268:string[])
                n168 = Match First String(2:w268, 3:w272) -> (0:w267:i32)  [unwired: 1 out]
                n169 = property on="Test Ring" class="Ring (strict)"("Value"=w267, "Strings []"=w268) -> ()  [unwired: 2 in, 2 out]
                n170 = property on="Test Ring" class="Ring (strict)"("Visible"=TRUE) -> ()  [unwired: 2 in, 2 out]
                n171 = property on="Test Slider" class="Slide (strict)"("Visible"=FALSE) -> ()  [unwired: 2 in, 2 out]
              }
              frame "Exposure  **" {
                n172 = Index Array(array=w279, index=2) -> (element=w280:cluster{string[]})
                n173 = call <vilib>:"NT Read String.vi"("name"=w282) -> ("value"=w281:string)  [unwired: 8 in, 2 out]
                n174 = Unbundle(w280) -> (w276:string[])
                n175 = Match First String(2:w276, 3:w281) -> (0:w277:i32)  [unwired: 1 out]
                n176 = property on="Test Ring" class="Ring (strict)"("Value"=w277, "Strings []"=w276) -> ()  [unwired: 2 in, 2 out]
                n177 = property on="Test Ring" class="Ring (strict)"("Visible"=TRUE) -> ()  [unwired: 2 in, 2 out]
                n178 = property on="Test Slider" class="Slide (strict)"("Visible"=FALSE) -> ()  [unwired: 2 in, 2 out]
              }
              frame "Exposure Priority  **" {
                n179 = Index Array(array=w288, index=3) -> (element=w289:cluster{string[]})
                n180 = call <vilib>:"NT Read String.vi"("name"=w291) -> ("value"=w290:string)  [unwired: 8 in, 2 out]
                n181 = Unbundle(w289) -> (w285:string[])
                n182 = Match First String(2:w285, 3:w290) -> (0:w286:i32)  [unwired: 1 out]
                n183 = property on="Test Ring" class="Ring (strict)"("Value"=w286, "Strings []"=w285) -> ()  [unwired: 2 in, 2 out]
                n184 = property on="Test Ring" class="Ring (strict)"("Visible"=TRUE) -> ()  [unwired: 2 in, 2 out]
                n185 = property on="Test Slider" class="Slide (strict)"("Visible"=FALSE) -> ()  [unwired: 2 in, 2 out]
              }
              frame "Color Enable  **" {
                n186 = Index Array(array=w297, index=4) -> (element=w298:cluster{string[]})
                n187 = call <vilib>:"NT Read String.vi"("name"=w300) -> ("value"=w299:string)  [unwired: 8 in, 2 out]
                n188 = Unbundle(w298) -> (w294:string[])
                n189 = Match First String(2:w294, 3:w299) -> (0:w295:i32)  [unwired: 1 out]
                n190 = property on="Test Ring" class="Ring (strict)"("Value"=w295, "Strings []"=w294) -> ()  [unwired: 2 in, 2 out]
                n191 = property on="Test Ring" class="Ring (strict)"("Visible"=TRUE) -> ()  [unwired: 2 in, 2 out]
                n192 = property on="Test Slider" class="Slide (strict)"("Visible"=FALSE) -> ()  [unwired: 2 in, 2 out]
              }
              frame Default {
                n193 = property on="Test Ring" class="Ring (strict)"("Visible"=FALSE) -> ()  [unwired: 2 in, 2 out]
                n194 = property on="Test Slider" class="Slide (strict)"("Visible"=FALSE) -> ()  [unwired: 2 in, 2 out]
              }
              frame "Brightness  **", "Color Level  **", "Compression  **", "FPS  **", "Sharpness  **" {
                n195 = call <vilib>:"NT Read Number.vi"("name"=w306) -> ("value"=w305:dbl)  [unwired: 8 in, 2 out]
                n196 = local write "Test Slider"(w305) -> ()
                n197 = property on="Test Slider" class="Slide (strict)"("Visible"=TRUE, "Scale.Maximum"=100.0 ("Scale.Range:Maximum")) -> ()  [unwired: 2 in, 2 out]
                n198 = property on="Test Ring" class="Ring (strict)"("Visible"=FALSE) -> ()  [unwired: 2 in, 2 out]
              }
            }
          }
        }
        n199 = property on="Progress" class="Clust (strict)"("Visible"=FALSE) -> ()  [unwired: 2 in, 2 out]
      }
      event "Test Name": Mouse Enter {
        # "Populate the ring with the list of tests"
        n200 = event-data() -> ()  [unwired: 1 in, 1 out]
        n201 = call <vilib>:"NT Read String Array.vi"("name"="TestMode/TestList" ("Name")) -> ("value"=w313:string[])  [unwired: 8 in, 2 out]
        n202 = Build Array (concatenate)("Select the test to run...", w313) -> (w312:string[])
        n203 = property on="Test Name" class="Ring (strict)"("Strings []"=w312) -> ()  [unwired: 2 in, 2 out]
      }
      event "Test Name": Value Change {
        w314 = FALSE ("Visible")
        # "Tell the robot the test name to run"
        n204 = event-data() -> ("NewVal"=w318:u16)  [unwired: 1 in]
        n205 = property on="Test Name" class="Ring (strict)"() -> ("Strings []"=w319:string[])  [unwired: 2 in, 2 out]
        n206 = local write "Progress"(T6 {"Test Progress"=0, "Test Progress Text"=""} ("Progress")) -> ()
        n207 = Index Array(array=w319, index=w318) -> (element=w317:string)
        n208 = call <vilib>:"NT Write String.vi"("value"=w317, "name"="TestMode/TestName" ("Name")) -> ()  [unwired: 9 in, 1 out]
        n209 = property on="Progress" class="Clust (strict)"("Visible"=TRUE) -> ()  [unwired: 2 in, 2 out]
        n210 = property on="Motor" class="Clust (strict)"("Visible"=w314) -> ()  [unwired: 2 in, 2 out]
        n211 = property on="Test Slider" class="Slide (strict)"("Visible"=w314) -> ()  [unwired: 2 in, 2 out]
        n212 = property on="On/Off" class="Bool (strict)"("Visible"=w314) -> ()  [unwired: 2 in, 2 out]
        n213 = property on="Rev/Fwd" class="Clust (strict)"("Visible"=w314) -> ()  [unwired: 2 in, 2 out]
        n214 = property on="Test Ring" class="Ring (strict)"("Visible"=w314) -> ()  [unwired: 2 in, 2 out]
      }
      event "Select Auto": Mouse Enter {
        # "Populate the combo box with the list of autonomous options"
        n215 = event-data() -> ()  [unwired: 1 in, 1 out]
        n216 = call <vilib>:"NT Read String Array.vi"("name"="Auto List" ("Name")) -> ("value"=w321:string[])  [unwired: 8 in, 2 out]
        n217 = property on="Select Auto" class="CmbBox"("Strings[]"=w321) -> ()  [unwired: 2 in, 2 out]
      }
      event "Select Auto": Value Change {
        # "User modified the Auto Selection. Write to NT variable so robot knows."
        n218 = event-data() -> ("NewVal"=w323:string)  [unwired: 1 in]
        n219 = call <vilib>:"NT Write String.vi"("value"=w323, "name"="Auto Selector" ("Name")) -> ()  [unwired: 9 in, 1 out]
      }
      event "CheckList": Double Click {
        # "Shift clears all"
        # "Update symbols on the listbox"
        n220 = event-data() -> ("PlatMods.Shift"=w325:bool, "Row"=w327:i32)  [unwired: 1 in]
        n221 = case shown="True" w325 {
          tunnel: w327 -> [w331 _]
          tunnel: 1 -> [w330 _]
          frame False {
            n222 = property on="CheckList" class="LstBox (strict)"() -> ("Item Symbols"=w329:i32[])  [unwired: 2 in, 2 out]
            n223 = Replace Array Subset(array=w329, new element=w330, index=w331) -> (w328:i32[])
            n224 = property on="CheckList" class="LstBox (strict)"("Item Symbols"=w328) -> ()  [unwired: 2 in, 2 out]
          }
          frame True {
            w332 = 0 ("Top Row")
            n225 = property on="CheckList" class="LstBox (strict)"() -> ("Number of Rows"=w334:u32)  [unwired: 2 in, 2 out]
            n226 = Initialize Array(0, w334) -> (w333:i32[])
            n227 = property on="CheckList" class="LstBox (strict)"("Top Row"=w332, "Value"=w332, "Item Symbols"=w333) -> ()  [unwired: 2 in, 2 out]
          }
        }
      }
      event "CheckList": Key Down {
        # "Update symbols on the listbox\nLeft and right keys check and uncheck"
        n228 = event-data() -> ("VKey"=w337:T22)  [unwired: 1 in]
        n229 = case shown="\"Left\", \"Right\"" w337 {
          selector: w337 -> [w342 _]
          tunnel: eventvkey."Left" ("VKey") -> [w340 _]
          frame "Left", "Right" {
            n230 = Equal?(x=w340, y=w342) -> (x = y?=w341:bool)
            n231 = Select(t=0, s=w341, f=1) -> (s? t:f=w343:i32)
            n232 = property on="CheckList" class="LstBox (strict)"() -> ("Item Symbols"=w346:i32[])  [unwired: 2 in, 2 out]
            n233 = Replace Array Subset(array=w346, new element=w343, index="CheckList") -> (w345:i32[])
            n234 = property on="CheckList" class="LstBox (strict)"("Item Symbols"=w345) -> ()  [unwired: 2 in, 2 out]
          }
          frame Default {
          }
        }
      }
      event "Motor.Enable": Value Change {
        # "When the test mode otor enable helper is set, update that\ntree row item's value"
        n235 = event-data() -> ("NewVal"=w351:bool)  [unwired: 1 in]
        n236 = Unbundle("Motor") -> ("Value"=w350:dbl)  [unwired: 1 out]
        n237 = Select(t=w350, s=w351, f=0.0) -> (s? t:f=w348:dbl)
        n238 = call <vilib>:"NT Write Number.vi"("value"=w348, "name"=w347) -> ()  [unwired: 9 in, 1 out]
      }
      event "Test Slider": Value Change {
        # "When the test mode slider helper is set, update that\ntree row item's value"
        n239 = event-data() -> ("NewVal"=w353:dbl)  [unwired: 1 in]
        n240 = call <vilib>:"NT Write Number.vi"("value"=w353, "name"=w354) -> ()  [unwired: 9 in, 1 out]
      }
      event "On/Off": Value Change {
        # "When the test mode on/off helper value is set, update that\ntree row item's value"
        n241 = event-data() -> ("NewVal"=w357:bool)  [unwired: 1 in]
        n242 = Boolean To (0,1)(Boolean=w357) -> (0, 1=w356:i16)
        n243 = call <vilib>:"NT Write Number.vi"("value"=w356, "name"=w355) -> ()  [unwired: 9 in, 1 out]
      }
      event "Rev/Fwd": Value Change {
        # "When the test mode helper value for relays is set, update that\ntree row item's value"
        n244 = event-data() -> ("NewVal.Forward"=w364:bool, "NewVal.Reverse"=w363:bool)  [unwired: 1 in]
        n245 = Boolean To (0,1)(Boolean=w364) -> (0, 1=w360:i16)
        n246 = Boolean To (0,1)(Boolean=w363) -> (0, 1=w362:i16)
        n247 = Negate(x=w362) -> (-x=w361:i16)
        n248 = Add(x=w360, y=w361) -> (x+y=w359:i16)
        n249 = call <vilib>:"NT Write Number.vi"("value"=w359, "name"=w358) -> ()  [unwired: 9 in, 1 out]
      }
      event "Test Ring": Value Change {
        # "When a test mode helper value is selected from the ring,\nset the tree item's variable to the string value"
        n250 = event-data() -> ("NewVal"=w367:u16)  [unwired: 1 in]
        n251 = property on="Test Ring" class="Ring (strict)"() -> ("Strings []"=w368:string[])  [unwired: 2 in, 2 out]
        n252 = Index Array(array=w368, index=w367) -> (element=w366:string)
        n253 = call <vilib>:"NT Write String.vi"("value"=w366, "name"=w365) -> ()  [unwired: 9 in, 1 out]
      }
      event "Rec Mode": Value Change {
        # "Update globals for recording mode and path to read log from.\nClear when logging and let NetworkTables set path for vision to\nuse."
        n254 = event-data() -> ("NewVal"=w377:enum32{"Stop", "Record", "Playback"})  [unwired: 1 in]
        n255 = global write "WPI_DashboardLogging Global.vi" "Logging Filename"(path "") -> ()
        n256 = global write "WPI_DashboardLogging Global.vi" "Recording"(w377) -> ()
        n257 = case shown="\"Playback\"" w377 {
          tunnel: w376 -> [_ w379 w387]
          tunnel: [_ _ w386] -> w374
          tunnel: [_ _ w385] -> _
          tunnel: w372 -> [_ _ w383]
          tunnel: cluster{i32, i32} {-250, 170} -> [_ _ w382]
          tunnel: [_ _ T23 {"Image Size"=TRUE, "Image Type"=TRUE, "Pixel Value"=TRUE, "ROI Information"=TRUE, "Zoom Factor"=FALSE} ("Image Information Shown:All Elements")] -> w369
          tunnel: [_ _ TRUE ("Zoom Factor")] -> w370
          frame Default {
          }
          frame "Stop", "Record" {
            # "Place Window too"
            n258 = invoke class="VI" method="FP.Close"(reference=w379) -> (reference out=w378:refnum<vi>)  [unwired: 2 in, 2 out]
            n259 = invoke class="VI" method="Abort VI"(reference=w378) -> ()  [unwired: 2 in, 3 out]
          }
          frame "Playback" {
            n260 = call "Open Playback Panel.vi"("Offset"=w382, "DB VI Ref"=w383, "Playback in"=w387) -> ("Playback out"=w384:refnum<vi>)  [unwired: 8 in]
            n261 = register-events(w384) -> (reference out=w386:refnum<event-registration>, error out=w385:errorcluster)  [unwired: 2 in]
          }
        }
        n262 = property on="Camera Image Right" class="ImageControl"("Image Information Shown"=w369, "Image Information Visible"=w370) -> ()  [unwired: 2 in, 2 out]
        n263 = property on="Camera Image" class="ImageControl"("Image Information Shown"=w369, "Image Information Visible"=w370) -> ()  [unwired: 2 in, 2 out]
        n264 = call <vilib>:"WPI_DashboardNT Log FieldName Cache.vi"("Operation"=enum16{"Lookup/Add", "Index", "Clear"}."Clear") -> ()  [unwired: 8 in, 3 out]
      }
      event Panel Close {
        w388 = enum32{"Stop", "Record", "Playback"}."Stop" ("Rec Mode")
        # "Playback window has been closed, abort"
        n265 = event-data() -> ()  [unwired: 1 in, 4 out]
        n266 = local write "Rec Mode"(w388) -> ()
        n267 = global write "WPI_DashboardLogging Global.vi" "Recording"(w388) -> ()
      }
      event Panel Close {
        # "Abort playback window and ourself"
        n268 = event-data() -> ()  [unwired: 1 in, 4 out]
        n269 = invoke class="VI" method="FP.Close"(reference=w391) -> (reference out=w390:refnum<vi>)  [unwired: 2 in, 2 out]
        n270 = invoke class="VI" method="Abort VI"(reference=w390) -> (error out=w389:errorcluster)  [unwired: 2 in, 2 out]
        n271 = invoke class="VI" method="Abort VI"(error in=w389) -> ()  [unwired: 2 in, 3 out]
      }
      event "Tree": Double Click {
        n272 = event-data() -> ("PlatMods"=w397:T25, "Tag"=w394:string)  [unwired: 1 in]
        n273 = Unbundle(w397) -> ("Shift"=w396:bool)  [unwired: 4 out]
        n274 = String Subset(string=w394, length (rest)=1 ("length (rest)")) -> (substring=w393:string)  [unwired: 1 in]
        n275 = Not(x=w396) -> (.not. x?=w395:bool)
        n276 = case shown="\"/\"" w393 {
          tunnel: w394 -> [_ w399]
          tunnel: w395 -> [_ w398]
          frame Default {
          }
          frame "/" {
            n277 = call <vilib>:"NT Update Persistence.vi"("Persistence"=w398, "Name"=w399) -> ()  [unwired: 9 in, 1 out]
          }
        }
      }
    }
  }
  n278 = while {
    tunnel: w54 -> [w401]
    i -> [w404]
    stop <- FALSE stop-if-true
    n279 = Wait (ms)(milliseconds to wait=u32 100) -> ()  [unwired: 1 out]
    n280 = case shown="\"Playback\"" "Rec Mode" {
      tunnel: w404 -> [_ _ w419]
      tunnel: [u32 2829099 ("Base Color") u32 11141120 ("Target Color") w408] -> w400
      frame "Stop", Default {
        # "Reset the color, extra updates don't cost much"
      }
      frame "Record" {
      }
      frame "Playback" {
        # "Playback"
        n281 = Quotient & Remainder(x=w419, y=u32 50 ("milliseconds to wait")) -> (x-y*floor(x/y)=w415:u32)  [unwired: 1 out]
        n282 = Divide(x=w415, y=u32 50 ("milliseconds to wait")) -> (x/y=w412:dbl)
        n283 = Multiply(x=6.283185307179586, y=w412) -> (x*y=w417:dbl)
        n284 = Sine(x=w417) -> (sin(x)=w416:dbl)
        n285 = Absolute Value(x=w416) -> (abs(x)=w409:dbl)
        n286 = call "Interpolate RGB Color.vi"("Proportion"=w409, "Target Color"=u32 30976, "Base Color"=u32 2829099) -> ("Result Color"=w408:u32)  [unwired: 8 in]
      }
    }
    n287 = property class="Pane"(reference=w401, "PaneColor"=w400) -> ()  [unwired: 1 in, 2 out]
  }
  n288 = local write "Dashboard Tab"(T2."Drive" ("Dashboard Tab")) -> ()
  n289 = property on="On/Off" class="Bool (strict)"("Visible"=w27) -> ()  [unwired: 2 in, 2 out]
  n290 = property on="Motor" class="Clust (strict)"("Visible"=w27) -> ()  [unwired: 2 in, 2 out]
  n291 = property on="Progress" class="Clust (strict)"("Visible"=w27) -> ()  [unwired: 2 in, 2 out]
  n292 = property on="Test Ring" class="Ring (strict)"("Visible"=w27) -> ()  [unwired: 2 in, 2 out]
  n293 = property on="Rev/Fwd" class="Clust (strict)"("Visible"=w27) -> ()  [unwired: 2 in, 2 out]
  n294 = while {
    tunnel: u16 1741 ("timeout ms (25000)") -> [w421]
    stop <- FALSE stop-if-true
    n295 = TCP Create Listener(10:w421) -> (0:w420:errorcluster, 3:w422:refnum<k5>)  [unwired: 4 in, 1 out]
    n296 = case shown="No Error" w420 {
      selector: w420 -> [w424 _]
      tunnel: w422 -> [w425 _]
      frame No Error {
        n297 = while {
          tunnel: w425 -> [w428]
          tunnel: w424 -> [w427]
          stop <- FALSE stop-if-true
          n298 = TCP Wait On Listener(8:w427, 11:w428) -> (0:w429:errorcluster, 4:w430:refnum<k5>)  [unwired: 2 in, 3 out]
          n299 = local write "TCP"(w430) -> ()
          n300 = case shown="Error" w429 {
            frame No Error {
            }
            frame Error {
              n301 = Wait (ms)(milliseconds to wait=u32 1000) -> ()  [unwired: 1 out]
            }
          }
        }
      }
      frame Error {
        n302 = Wait (ms)(milliseconds to wait=u32 1000) -> ()  [unwired: 1 out]
      }
    }
  }
  n303 = global write "WPI_DashboardLogging Global.vi" "Recording"(w49) -> ()
  n304 = local write "Rec Mode"(w49) -> ()
  n305 = call <vilib>:"NT Write String.vi"("value"="Select Auto", "name"="Auto Selector" ("Name")) -> ()  [unwired: 9 in, 1 out]
